vi "labviewTest.vi"() -> ()   [LabVIEW 2018]
uses:
  Program Files (x86)/National Instruments/LabVIEW 2018/examples/Connectivity/Python/support/PythonVersionsEnum.ctl
  PythonConfigGlobal.vi
panel:
  in  "matrix size":i32
  in  "matrix type":i32(ring)=1 items=["zeros", "단위"]
  out "ans":dbl[][](array[numeric])=[[1.0, 2.0], [3.0, 4.0]]
  out "Eigen values":cdb[](array[numeric]) caption="고유값"
  out "Eigen vectors":cdb[][](array[numeric])
  in  "matrix":dbl[][](array[numeric])=[[1.0, 2.0], [3.0, 4.0]]
  out "ans":dbl[][](array[numeric])=[[1.0, 2.0], [3.0, 4.0]]
  in  "matrix":dbl[][](array[numeric])=[[1.0, 2.0], [3.0, 4.0]]
  in  "matrix":dbl[][](array[numeric])=[[1.0, 2.0], [3.0, 4.0]]
  out "ans":dbl
  in  "a":dbl[][](array[numeric])=[[1.0, 1.0]]
  out "ans":dbl[][](array[numeric])=[[1.0], [1.0]]
  in  "b":dbl[][](array[numeric])=[[1.0, 1.0], [1.0, 1.0]]
  in  "a":dbl[][](array[numeric])=[[1.0, 1.0]]
  out "ans":dbl[][](array[numeric])=[[2.0, 2.0]]
  out "error out":errorcluster
  in  "error in (no error)":errorcluster
  in  "python version":T1=enum."3.6"
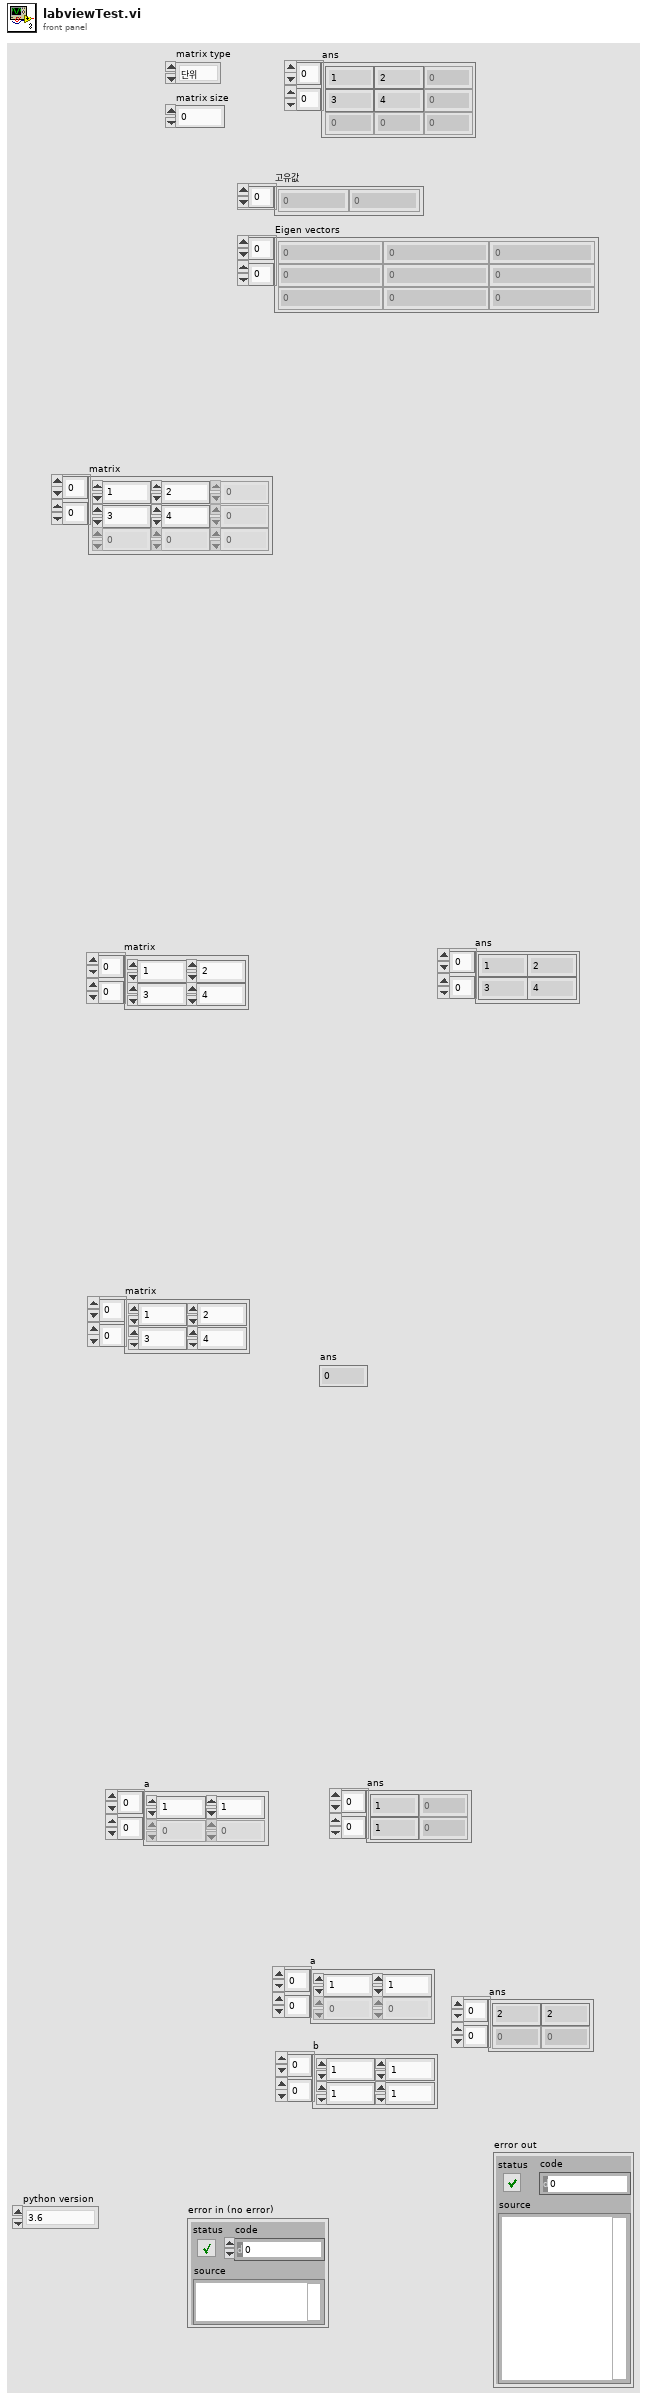
[diagram p1: front panel]
types:
  T1 = typedef "PythonVersionsEnum.ctl" = enum16{"2.7", "3.6"}
  T2 = cluster{"session out":refnum<k35>, "appended path":path}
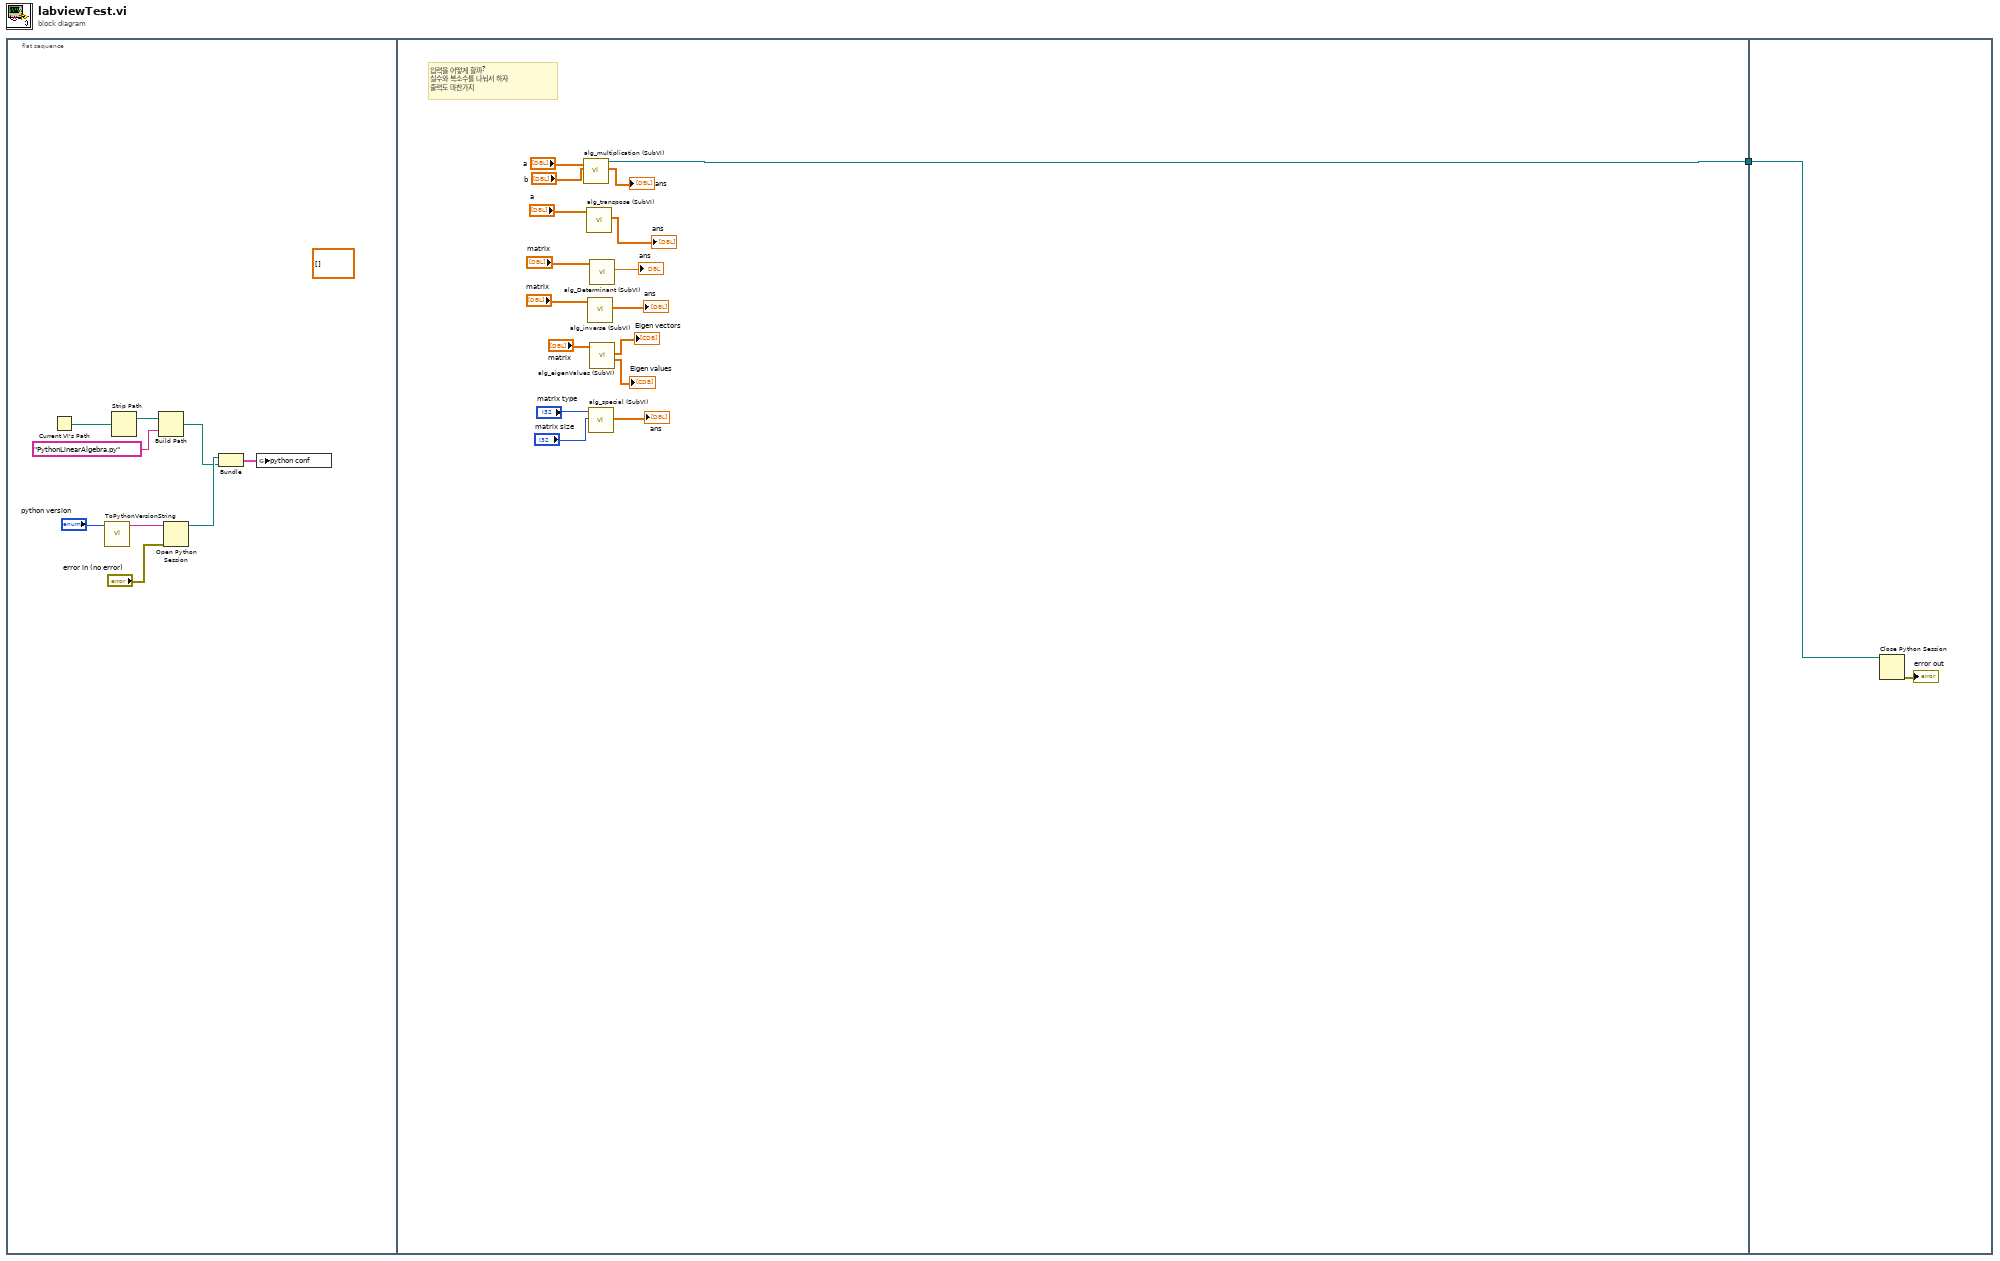
[diagram p0: block diagram]
diagram:
  n1 = flat-sequence {
    tunnel: [w23] -> w1
    tunnel: w1 -> [w27]
    frame #0 {
      (unwired) dbl[][] [] ("str1")
      n2 = Current VI's Path() -> (path=w6:path)
      n3 = call "ToPythonVersionString.vi"("python version"="python version") -> ("python version string"=w8:string)  [unwired: 10 in]
      n4 = Strip Path(path=w6) -> (stripped path=w7:path)  [unwired: 1 out]
      n5 = Build Path(base path=w7, name or relative path="PythonLinearAlgebra.py") -> (appended path=w9:path)
      n6 = Open Python Session(python version=w8, 3:"error in (no error)") -> (session out=w10:refnum<k35>)  [unwired: 1 in, 1 out]
      n7 = Bundle("session out"=w10, "appended path"=w9) -> (w2:T2)  [unwired: 1 in]
      n8 = global write "PythonConfigGlobal.vi" "python conf"(w2) -> ()
    }
    frame #1 {
      # "입력을 어떻게 할까?\n실수와 복소수를 나눠서 하자\n출력도 마찬가지"
      n9 = call "alg_multiplication (SubVI).vi"("b"="b", "a"="a") -> ("ans"=→"ans":dbl[][], "참조 번호 출력"=w23:refnum<k35>)  [unwired: 7 in, 1 out]
      n10 = call "alg_transpose (SubVI).vi"("matrix"="a") -> ("ans"=→"ans":dbl[][])  [unwired: 8 in, 2 out]
      n11 = call "alg_inverse (SubVI).vi"("matrix"="matrix") -> ("ans"=→"ans":dbl[][])  [unwired: 8 in, 2 out]
      n12 = call "alg_special (SubVI).vi"("matrix size"="matrix size", "matrix type"="matrix type") -> ("ans"=→"ans":dbl[][])  [unwired: 7 in, 2 out]
      n13 = call "alg_Determinant (SubVI).vi"("matrix"="matrix") -> ("ans"=→"ans":dbl)  [unwired: 8 in, 2 out]
      n14 = call "alg_eigenValues (SubVI).vi"("matrix"="matrix") -> ("Eigen values"=→"Eigen values":cdb[], "Eigen vectors"=→"Eigen vectors":cdb[][])  [unwired: 7 in, 2 out]
    }
    frame #2 {
      n15 = Close Python Session(session in=w27) -> (11:→"error out":errorcluster)  [unwired: 1 in]
    }
  }
